vi "Main.vi"(11 "Module Admin":refnum<class "Delacor_lib_QMH_Module Admin.lvclass">) -> ()   [LabVIEW 2020, in "UI.lvlib"]
doc: "This template is based off of the Queued Message Handler design pattern and the Queued Message Handler project template that ships with LabVIEW.\n\nThe main difference is that the queue is private to this module and communication between modules is performed via Broadcast and Request events.\n\nRequest events are wrapped in public API methods and are handled in the Event Handling Loop (EHL) of this VI. Any module can register for Broadcast events sent by this module. The EHL generates messages based on user interface actions.\n\nThe Message Handling Loop (MHL) processes messages generated by the EHL, or by other messages. The messages are string values, so new messages can be added easily to the Message Cases case structure in the MHL. Each message cluster can also provide an optional value for Message Data, which is a variant that can be converted to whatever message-specific data is required.\n_____\nBased on Delacor QMH Project Template 5.0.0.82."
uses:
  UI.lvlib
  <vilib>/Delacor/Delacor QMH/Libraries/Module Admin_class/Delacor_lib_QMH_Module Admin.lvclass
  Module Data--cluster.ctl
  Stop Argument--cluster.ctl
  <vilib>/Delacor/Delacor QMH/Libraries/Message Queue_class/Delacor_lib_QMH_Message Queue.lvclass/Delacor_lib_QMH_Message Queue.ctl
  <vilib>/Delacor/Delacor QMH/Libraries/Module Admin_class/Delacor_lib_QMH_Module Admin.lvclass/Delacor_lib_QMH_Module Admin.ctl
  <vilib>/Delacor/Delacor QMH/Libraries/Message Queue_class/Delacor_lib_QMH_Enqueue Message (Single).vi
  <vilib>/Delacor/Delacor QMH/Libraries/Module Admin_class/Delacor_lib_QMH_Get External Launch.vi
  <vilib>/Utility/error.llb/Error Cluster From Error Code.vi
  <vilib>/ErrorRing/Error Ring.xnode
  <vilib>/Delacor/Delacor QMH/Libraries/Message Queue_class/Delacor_lib_QMH_Message Queue.lvclass
  Acquisiton Oscar Template/Acquisiton Oscar Template.lvlib
  Config/Config.lvlib
  Logging/Logging.lvlib
panel:
  in  "Config":bool
  in  "Stop Acq":bool
  in  "Start Acq":bool
  out "error out":errorcluster
  out "Status":string
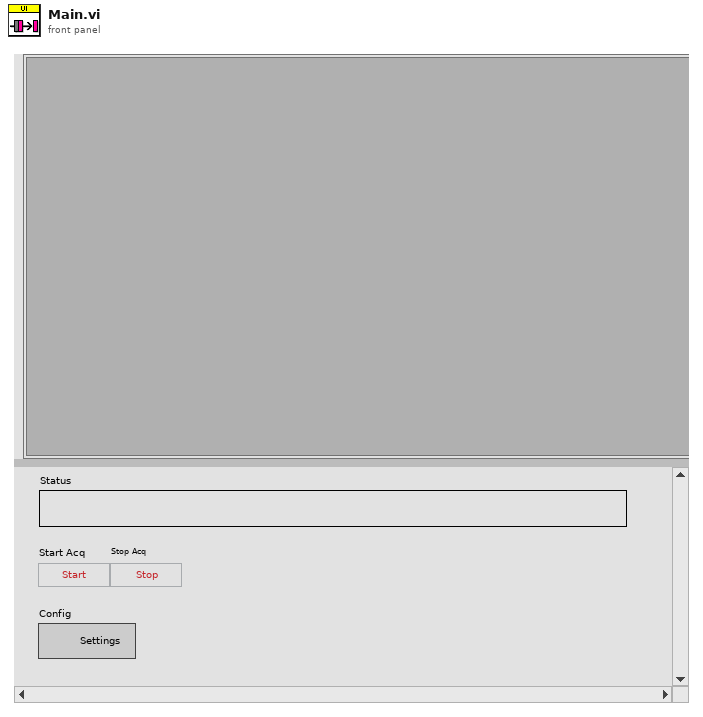
[diagram p1: front panel]
types:
  T1 = typedef "UI.lvlib/Request Events--cluster.ctl" = cluster{"Stop Module":refnum<user-event>, "Show Panel":refnum<user-event>, "Hide Panel":refnum<user-event>, "Get Module Execution Status":refnum<user-event>, "Show Diagram":refnum<user-event>}
  T2 = typedef "Acquisiton Oscar Template.lvlib/Broadcast Events--cluster.ctl" = cluster{"Module Did Init":refnum<user-event>, "Status Updated":refnum<user-event>, "Error Reported":refnum<user-event>, "Module Did Stop":refnum<user-event>, "Update Module Execution Status":refnum<user-event>}
  T3 = typedef "Config.lvlib/Broadcast Events--cluster.ctl" = cluster{"Module Did Init":refnum<user-event>, "Status Updated":refnum<user-event>, "Error Reported":refnum<user-event>, "Module Did Stop":refnum<user-event>, "Update Module Execution Status":refnum<user-event>}
  T4 = typedef "Logging.lvlib/Broadcast Events--cluster.ctl" = cluster{"Module Did Init":refnum<user-event>, "Status Updated":refnum<user-event>, "Error Reported":refnum<user-event>, "Module Did Stop":refnum<user-event>, "Update Module Execution Status":refnum<user-event>}
  T5 = typedef "UI.lvlib/Module Data--cluster.ctl" = cluster{"Status":string}
  T6 = enum32{"invalid lock state", "Not Locked", "Locked (No Password)", "Password-protected"}
  T7 = typedef "UI.lvlib/Stop Argument--cluster.ctl" = cluster{"Origin":string, "Exit via Stop Module Req?":bool, "Wait for Module to stop?":bool}
  T8 = enum32{"Invalid", "Standard", "Closed", "Hidden", "Minimized", "Maximized"}
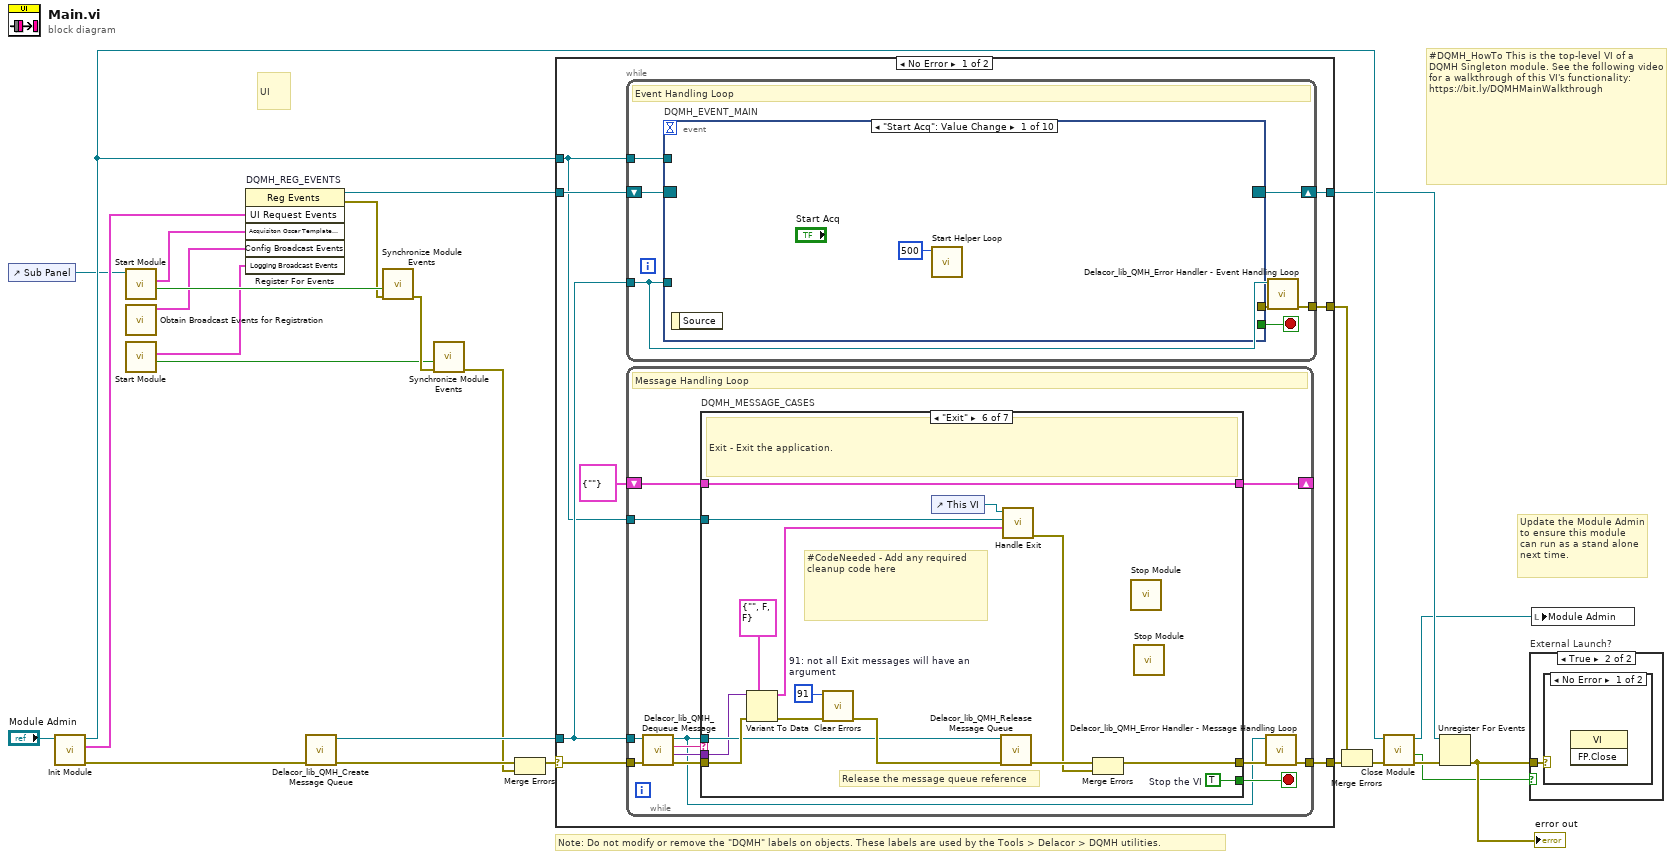
[diagram p0: block diagram]
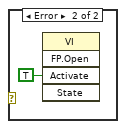
[diagram p3: hidden frame]
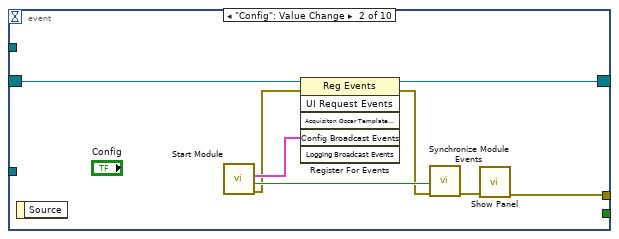
[diagram p4: hidden frame]
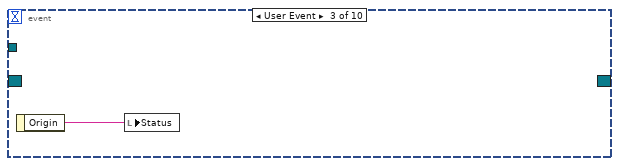
[diagram p5: hidden frame]
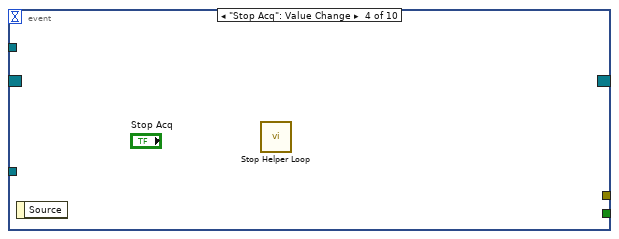
[diagram p6: hidden frame]
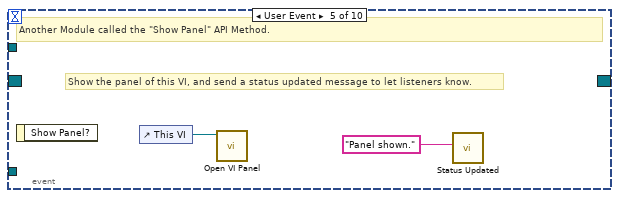
[diagram p7: hidden frame]
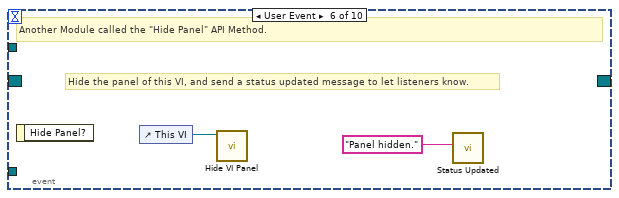
[diagram p8: hidden frame]
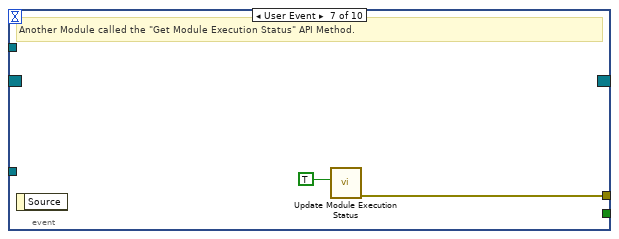
[diagram p9: hidden frame]
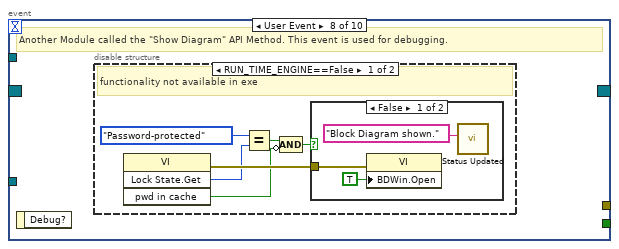
[diagram p10: hidden frame]
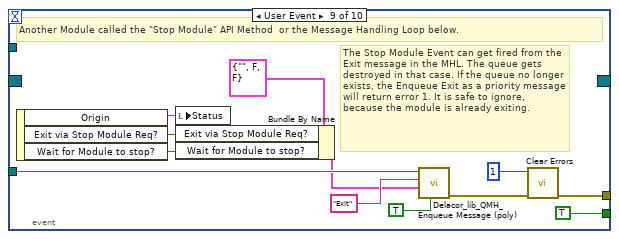
[diagram p13: hidden frame]
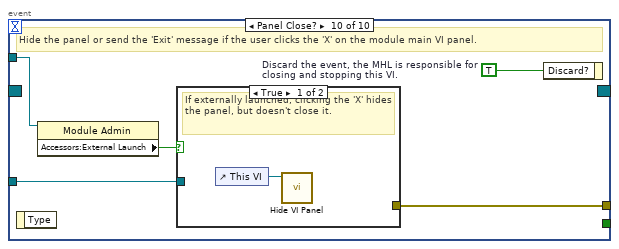
[diagram p14: hidden frame]
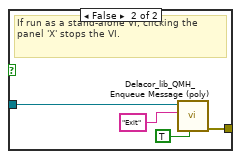
[diagram p15: hidden frame]
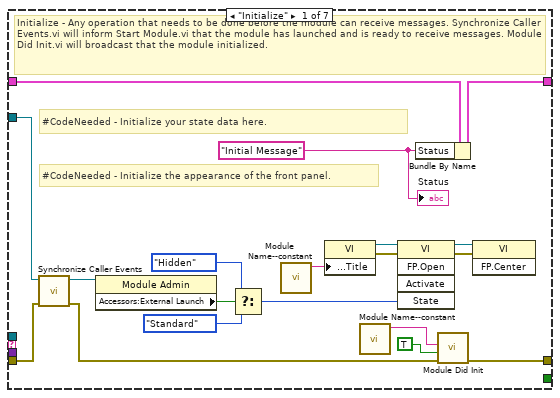
[diagram p16: hidden frame]
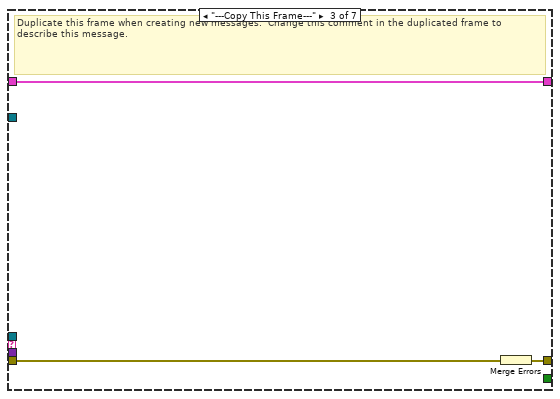
[diagram p18: hidden frame]
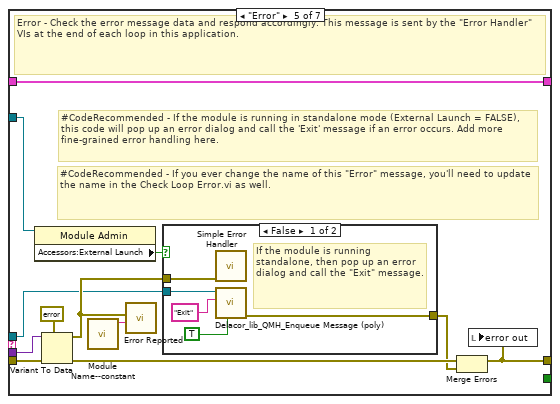
[diagram p20: hidden frame]
diagram:
  # "UI"
  # "#DQMH_HowTo This is the top-level VI of a DQMH Singleton module. See the following video for a walkthrough of this VI's functionality: https://bit.ly/DQMHMainWalkthrough"
  # "Note: Do not modify or remove the \"DQMH\" labels on objects. These labels are used by the Tools > Delacor > DQMH utilities."
  # "Update the Module Admin to ensure this module can run as a stand alone next time."
  n1 = control-ref of="Sub Panel"() -> (w6:refnum<vi>)
  n2 = call "Init Module.vi"("Singleton Module Admin in"="Module Admin") -> ("error out"=w24:errorcluster, "UI Request Events"=w14:T1, "Singleton Module Admin out"=w17:refnum<class "Delacor_lib_QMH_Module Admin.lvclass">)  [unwired: 8 in]
  n3 = call "Start Module.vi"("Sub Panel"=w6) -> ("Wait for Event Sync?"=w8:bool, "Acquisiton Oscar Template Broadcast Events"=w9:T2)  [unwired: 7 in, 2 out]
  n4 = call "Obtain Broadcast Events for Registration.vi"() -> ("Config Broadcast Events"=w5:T3)  [unwired: 9 in, 2 out]
  n5 = call "Start Module.vi"() -> ("Wait for Event Sync?"=w1:bool, "Logging Broadcast Events"=w2:T4)  [unwired: 8 in, 2 out]
  n6 = register-events "DQMH_REG_EVENTS"(w14, w9, w5, w2) -> (reference out=w15:refnum<event-registration>, error out=w7:errorcluster)  [unwired: 2 in]
  n7 = call <vilib>:"Delacor_lib_QMH_Create Message Queue.vi"("error in (no error)"=w24) -> ("error out"=w19:errorcluster, "Message Queue"=w13:refnum<class "Delacor_lib_QMH_Message Queue.lvclass">)  [unwired: 9 in]
  n8 = call "Synchronize Module Events.vi"("error in (no error)"=w7, "Wait for Event Sync?"=w8) -> ("error out"=w4:errorcluster)  [unwired: 9 in]
  n9 = call "Synchronize Module Events.vi"("error in (no error)"=w4, "Wait for Event Sync?"=w1) -> ("error out"=w3:errorcluster)  [unwired: 9 in]
  n10 = Merge Errors(w19, w3) -> (w18:errorcluster)
  n11 = case shown="No Error" w18 {
    selector: w18 -> [w31 w174]
    tunnel: [w33 w173] -> w25
    tunnel: [w30 w179] -> w16
    tunnel: w15 -> [w28 w179]
    tunnel: w13 -> [w27 w172]
    tunnel: [w32 _] -> w22
    tunnel: w17 -> [w26 w175]
    frame No Error {
      n12 = while {
        tunnel: w27 -> [w34]
        shift-right: [w37] -> w30
        shift-left: w28 -> [w38]
        tunnel: [w39] -> w32
        tunnel: w26 -> [w35]
        stop <- w36 stop-if-true
        # "Event Handling Loop"
        n13 = event "DQMH_EVENT_MAIN" shown="[0] \"Start Acq\": Value Change" {
          selector: w38 -> [_ w49 _ _ _ _ _ _ _ _]
          dyn-events: [_ w44 _ _ _ _ _ _ _ _] -> w37
          timeout: _ -> [_ _ _ _ _ _ _ _ _ _]
          tunnel: [_ _ _ _ _ _ _ _ TRUE ("Discard?") _] -> w36
          tunnel: w34 -> [_ _ _ _ _ _ _ _ w73 w80]
          tunnel: [_ w42 _ _ _ _ w56 _ w76 w82] -> w40
          tunnel: w35 -> [_ _ _ _ _ _ _ _ _ w79]
          event "Start Acq": Value Change {
            n14 = event-data() -> ()  [unwired: 1 in, 1 out]
            n15 = call "Start Helper Loop.vi"("Delay Timeout"=500) -> ()  [unwired: 10 in, 1 out]
          }
          event "Config": Value Change {
            n16 = event-data() -> ()  [unwired: 1 in, 1 out]
            n17 = call "Start Module.vi"() -> ("error out"=w46:errorcluster, "Wait for Event Sync?"=w47:bool, "Config Broadcast Events"=w48:T3)  [unwired: 8 in, 1 out]
            n18 = register-events(reference=w49, error in=w46, w48) -> (reference out=w44:refnum<event-registration>, error out=w45:errorcluster)  [unwired: 3 in]
            n19 = call "Synchronize Module Events.vi"("error in (no error)"=w45, "Wait for Event Sync?"=w47) -> ("error out"=w43:errorcluster)  [unwired: 9 in]
            n20 = call "Show Panel.vi"("error in (no error)"=w43) -> ("error out"=w42:errorcluster)  [unwired: 10 in]
          }
          event User Event {
            n21 = event-data() -> ("Origin"=w50:string)  [unwired: 1 in]
            n22 = local write "Status"(w50) -> ()
          }
          event "Stop Acq": Value Change {
            n23 = event-data() -> ()  [unwired: 1 in, 1 out]
            n24 = call "Stop Helper Loop.vi"() -> ()  [unwired: 11 in, 1 out]
          }
          event User Event {
            # "Show the panel of this VI, and send a status updated message to let listeners know."
            # "Another Module called the \"Show Panel\" API Method."
            n25 = event-data() -> ()  [unwired: 1 in, 1 out]
            n26 = control-ref of="This VI"() -> (w52:refnum<vi>)
            n27 = call "Open VI Panel.vi"("VI"=w52) -> ()  [unwired: 10 in, 1 out]
            n28 = call "Status Updated.vi"("Status"="Panel shown." ("format string")) -> ()  [unwired: 10 in, 1 out]
          }
          event User Event {
            # "Hide the panel of this VI, and send a status updated message to let listeners know."
            # "Another Module called the \"Hide Panel\" API Method."
            n29 = event-data() -> ()  [unwired: 1 in, 1 out]
            n30 = control-ref of="This VI"() -> (w54:refnum<vi>)
            n31 = call "Hide VI Panel.vi"("VI"=w54) -> ()  [unwired: 10 in, 1 out]
            n32 = call "Status Updated.vi"("Status"="Panel hidden." ("format string")) -> ()  [unwired: 10 in, 1 out]
          }
          event User Event {
            # "Another Module called the \"Get Module Execution Status\" API Method."
            n33 = event-data() -> ()  [unwired: 1 in, 1 out]
            n34 = call "Update Module Execution Status.vi"("Running?"=TRUE) -> ("error out"=w56:errorcluster)  [unwired: 10 in]
          }
          event User Event {
            # "Another Module called the \"Show Diagram\" API Method. This event is used for debugging."
            n35 = event-data() -> ()  [unwired: 1 in, 1 out]
            n36 = disable-structure shown="RUN_TIME_ENGINE==False" {
              frame condition #0 (active) {
                # "functionality not available in exe"
                n37 = invoke class="VI" method="Lock State.Get"() -> (error out=w62:errorcluster, "Get Lock State"=w61:T6, "pwd in cache"=w58:bool)  [unwired: 4 in, 1 out]
                n38 = Equal?(x=T6."Password-protected", y=w61) -> (x = y?=w59:bool)
                n39 = Compound Arithmetic op=AND(w59, invert w58) -> (w57:bool)
                n40 = case shown="False" w57 {
                  tunnel: w62 -> [w65 _]
                  frame False {
                    n41 = property class="VI"(error in=w65, "BDWin.Open"=TRUE ("Block Diagram Window:Open")) -> ()  [unwired: 1 in, 2 out]
                    n42 = call "Status Updated.vi"("Status"="Block Diagram shown." ("format string")) -> ()  [unwired: 10 in, 1 out]
                  }
                  frame True {
                    # "Password-protected VI, and the password is not in the cache. Do not show the diagram."
                  }
                }
              }
              frame condition #1 {
              }
            }
          }
          event User Event {
            # "The Stop Module Event can get fired from the Exit message in the MHL. The queue gets destroyed in that case. If the queue no longer exists, the Enqueue Exit as a priority message will return error 1. It is safe to ignore, because the module is already exiting."
            # "Another Module called the \"Stop Module\" API Method  or the Message Handling Loop below."
            n43 = event-data() -> ("Origin"=w72:string, "Exit via Stop Module Req?"=w68:bool, "Wait for Module to stop?"=w67:bool)  [unwired: 1 in]
            n44 = local write "Status"(w72) -> ()
            n45 = Bundle By Name(cluster=T7 {"Origin"="", "Exit via Stop Module Req?"=FALSE, "Wait for Module to stop?"=FALSE} ("Stop Argument"), "Exit via Stop Module Req?"=w68, "Wait for Module to stop?"=w67) -> (w66:T7)
            n46 = call-poly <vilib>:"Delacor_lib_QMH_Enqueue Message (poly).vi"("Priority Message? (F)"=TRUE, "Message Data"=w66, "Message"="Exit", "Message Queue in"=w73) -> ("error out"=w77:errorcluster)  [unwired: 6 in, 1 out]
            n47 = call <vilib>:"Clear Errors.vi"("error in (no error)"=w77, "specific error code to clear (0: all)"=1) -> ("error out"=w76:errorcluster)  [unwired: 4 in, 1 out]
          }
          event Panel Close? {
            w81 = TRUE  # Discard the event, the MHL is responsible for closing and stopping this VI.
            # "Hide the panel or send the 'Exit' message if the user clicks the 'X' on the module main VI panel."
            n48 = event-data() -> ()  [unwired: 1 in, 1 out]
            n49 = property class="Module Admin"(reference=w79) -> ("Accessors:External Launch"=w78:bool)  [unwired: 1 in, 2 out]
            n50 = case shown="True" w78 {
              tunnel: w80 -> [_ w86]
              tunnel: [_ w87] -> w82
              frame True {
                # "If externally launched, clicking the 'X' hides the panel, but doesn't close it."
                n51 = control-ref of="This VI"() -> (w83:refnum<vi>)
                n52 = call "Hide VI Panel.vi"("VI"=w83) -> ()  [unwired: 10 in, 1 out]
              }
              frame False {
                # "If run as a stand-alone VI, clicking the panel 'X' stops the VI."
                n53 = call-poly <vilib>:"Delacor_lib_QMH_Enqueue Message (poly).vi"("Priority Message? (F)"=TRUE, "Message"="Exit", "Message Queue in"=w86) -> ("error out"=w87:errorcluster)  [unwired: 7 in, 1 out]
              }
            }
            n54 = event-data("Discard?"=w81) -> ()  [unwired: 1 in, 1 out]
          }
        }
        n55 = call-dynamic "Delacor_lib_QMH_Error Handler - Event Handling Loop.vi"("error in (no error)"=w40, "Message Queue in"=w34) -> ("dup error in"=w39:errorcluster)  [unwired: 8 in, 1 out]
      }
      n56 = while {
        tunnel: w27 -> [w90]
        shift-right: [w94] -> _
        shift-left: T5 {"Status"=""} ("Data Cluster") -> [w95]
        tunnel: w31 -> [w98]
        tunnel: [w96] -> w33
        tunnel: w26 -> [w88]
        stop <- w93 stop-if-true
        # "Message Handling Loop"
        n57 = call-dynamic "Delacor_lib_QMH_Dequeue Message.vi"("error in (no error)"=w98, "Message Queue in"=w90) -> ("error out"=w97:errorcluster, "Message Data"=w91:variant, "Message"=w92:string, "Message Queue out"=w89:refnum<class "Delacor_lib_QMH_Message Queue.lvclass">)  [unwired: 6 in]
        n58 = case "DQMH_MESSAGE_CASES" shown="\"Exit\"" w92 {
          selector: w92 -> [_ _ _ _ _ _ w159]
          tunnel: w89 -> [_ _ _ _ w129 w151 _]
          tunnel: w97 -> [w116 w120 w123 w125 w136 w157 w161]
          tunnel: [w114 w120 w122 w125 w132 w154 w162] -> w99
          tunnel: w95 -> [w105 w119 w121 w124 w131 w150 w160]
          tunnel: [w104 w119 w121 w124 w131 w150 w160] -> w94
          tunnel: [_ _ _ _ _ w149 _] -> w93
          tunnel: w91 -> [_ _ _ _ w130 w148 _]
          tunnel: w88 -> [w106 _ _ _ w128 w143 _]
          frame "Initialize" {
            w100 = "Initial Message" ("Initial Message")
            # "#CodeNeeded - Initialize the appearance of the front panel."
            # "#CodeNeeded - Initialize your state data here."
            # "Initialize - Any operation that needs to be done before the module can receive messages. Synchronize Caller Events.vi will inform Start Module.vi that the module has launched and is ready to receive messages. Module Did Init.vi will broadcast that the module initialized."
            n59 = call "Synchronize Caller Events.vi"("error in (no error)"=w116, "Singleton Module Admin in"=w106) -> ("error out"=w115:errorcluster, "Singleton Module Admin out"=w101:refnum<class "Delacor_lib_QMH_Module Admin.lvclass">)  [unwired: 8 in]
            n60 = property class="Module Admin"(reference=w101) -> ("Accessors:External Launch"=w110:bool)  [unwired: 1 in, 2 out]
            n61 = Select(t=T8."Hidden" ("State"), s=w110, f=T8."Standard" ("State")) -> (s? t:f=w107:T8)
            n62 = call "Module Name--constant.vi"() -> ("Module Name"=w113:string)  [unwired: 11 in]
            n63 = property class="VI"("Front Panel.Title"=w113) -> (reference out=w112:refnum<vi>, error out=w118:errorcluster)  [unwired: 2 in]
            n64 = call "Module Name--constant.vi"() -> ("Module Name"=w102:string)  [unwired: 11 in]
            n65 = invoke class="VI" method="FP.Open"(reference=w112, error in=w118, "State"=w107) -> (reference out=w111:refnum<vi>, error out=w117:errorcluster)  [unwired: 2 in, 3 out]
            n66 = Bundle By Name(cluster=w105, "Status"=w100) -> (w104:T5)
            n67 = call "Module Did Init.vi"("error in (no error)"=w115, "Initialized?"=TRUE, "Origin"=w102) -> ("error out"=w114:errorcluster)  [unwired: 8 in]
            n68 = invoke class="VI" method="FP.Center"(reference=w111, error in=w117) -> ()  [unwired: 1 in, 3 out]
            "Status" <- w100
          }
          frame "--- Module Specific ---" {
            # "Separator -- The following cases handle messages specific to this Module."
          }
          frame "---Copy This Frame---" {
            # "Duplicate this frame when creating new messages.  Change this comment in the duplicated frame to describe this message."
            n69 = Merge Errors(w123) -> (w122:errorcluster)
          }
          frame "--- Exit and Error Handling---" {
            # "Separator - The following cases handle errors and exit messages."
          }
          frame "Error" {
            # "#CodeRecommended - If you ever change the name of this \"Error\" message, you'll need to update the name in the Check Loop Error.vi as well."
            # "#CodeRecommended - If the module is running in standalone mode (External Launch = FALSE), this code will pop up an error dialog and call the 'Exit' message if an error occurs. Add more fine-grained error handling here."
            # "Error - Check the error message data and respond accordingly. This message is sent by the \"Error Handler\" VIs at the end of each loop in this application."
            n70 = property class="Module Admin"(reference=w128) -> ("Accessors:External Launch"=w127:bool)  [unwired: 1 in, 2 out]
            n71 = Variant To Data(error in=w136, type=errorcluster {"status"=FALSE, "code"=0, "source"=""} ("error constant"), Variant=w130) -> (data=w137:errorcluster, error out=w134:errorcluster)
            n72 = call "Module Name--constant.vi"() -> ("Module Name"=w126:string)  [unwired: 11 in]
            n73 = call "Error Reported.vi"("Additional Information"=w126, "Error"=w137) -> ()  [unwired: 9 in, 1 out]
            n74 = case shown="False" w127 {
              tunnel: [w142 _] -> w133
              tunnel: w129 -> [w140 _]
              tunnel: w137 -> [w141 _]
              frame False {
                # "If the module is running standalone, then pop up an error dialog and call the \"Exit\" message."
                n75 = call <vilib>:"Simple Error Handler.vi"("error in (no error)"=w141) -> ()  [unwired: 4 in, 5 out]
                n76 = call-poly <vilib>:"Delacor_lib_QMH_Enqueue Message (poly).vi"("Priority Message? (F)"=TRUE, "Message"="Exit", "Message Queue in"=w140) -> ("error out"=w142:errorcluster)  [unwired: 7 in, 1 out]
              }
              frame True {
                # "If the module was launched externally, calling the Error Reported broadcast VI is the only action performed by the \"Error\" message. The module's caller can then process the error appropriately."
              }
            }
            n77 = Merge Errors(w134, w133) -> (w132:errorcluster)
            n78 = local write "error out"(w132) -> ()
          }
          frame "Exit" {
            w147 = 91  # 91: not all Exit messages will have an argument
            w149 = TRUE  # Stop the VI
            # "Release the message queue reference"
            # "#CodeNeeded - Add any required cleanup code here"
            # "Exit - Exit the application."
            n79 = Variant To Data(error in=w157, type=T7 {"Origin"="", "Exit via Stop Module Req?"=FALSE, "Wait for Module to stop?"=FALSE} ("Stop Argument"), Variant=w148) -> (data=w145:T7, error out=w153:errorcluster)
            n80 = call <vilib>:"Clear Errors.vi"("error in (no error)"=w153, "specific error code to clear (0: all)"=w147) -> ("error out"=w156:errorcluster)  [unwired: 4 in, 1 out]
            n81 = control-ref of="This VI"() -> (w144:refnum<vi>)
            n82 = call-dynamic "Delacor_lib_QMH_Release Message Queue.vi"("error in (no error)"=w156, "Message Queue"=w151) -> ("error out"=w155:errorcluster)  [unwired: 9 in]
            n83 = call "Handle Exit.vi"("Stop Argument"=w145, "Admin in"=w143, "VI reference"=w144) -> ("error out"=w152:errorcluster)  [unwired: 7 in, 1 out]
            n84 = Merge Errors(w155, w152) -> (w154:errorcluster)
            n85 = call "Stop Module.vi"() -> ()  [unwired: 11 in, 1 out]
            n86 = call "Stop Module.vi"() -> ()  [unwired: 11 in, 1 out]
          }
          frame Default {
            # "'Default' case only runs if there is a message that isn't defined in any of the other cases.  Output a programming error."
            n87 = call "Module Name--constant.vi"() -> ("Module Name"=w158:string)  [unwired: 11 in]
            n88 = xnode "Error Ring"("parameter 0"=w159, "parameter 1"=w158) -> ("error out"=w163:errorcluster)
            n89 = Merge Errors(w161, w163) -> (w162:errorcluster)
          }
        }
        n90 = call-dynamic "Delacor_lib_QMH_Error Handler - Message Handling Loop.vi"("error in (no error)"=w99, "Message Queue in"=w89) -> ("dup error in"=w96:errorcluster)  [unwired: 8 in, 1 out]
      }
    }
    frame Error {
      # "Synchronize Caller Events.vi will inform Start Module.vi that the module has launched and will let the code calling Start Module.vi register for broadcasts and would permit the caller receive the broadcast that an error occurred at launch time."
      n91 = call-dynamic "Delacor_lib_QMH_Release Message Queue.vi"("error in (no error)"=w174, "Message Queue"=w172) -> ("error out"=w173:errorcluster)  [unwired: 9 in]
      n92 = call "Synchronize Caller Events.vi"("Singleton Module Admin in"=w175) -> ("error out"=w180:errorcluster)  [unwired: 9 in, 1 out]
      n93 = call "Module Name--constant.vi"() -> ("Module Name"=w178:string)  [unwired: 11 in]
      n94 = Format Into String(format string="An error occurred during initialization. %s is no longer running.", w178) -> (resulting string=w176:string)  [unwired: 2 in, 1 out]
      n95 = Merge Errors(w173, w180) -> (w181:errorcluster)
      n96 = call "Error Reported.vi"("Additional Information"=w176, "Error"=w181) -> ()  [unwired: 9 in, 1 out]
    }
  }
  n97 = Merge Errors(w22, w25) -> (w21:errorcluster)
  n98 = call "Close Module.vi"("error in (no error)"=w21, "Module Admin in"=w17) -> ("error out"=w23:errorcluster, "External Launch"=w10:bool, "Module Admin out"=w11:refnum<class "Delacor_lib_QMH_Module Admin.lvclass">)  [unwired: 7 in]
  n99 = Unregister For Events(event registration refnum=w16, error in=w23) -> (error out=w20:errorcluster)
  "error out" <- w20
  n100 = case "External Launch?" shown="True" w10 {
    tunnel: w20 -> [_ w182]
    frame False {
    }
    frame True {
      n101 = case shown="No Error" w182 {
        frame No Error {
          n102 = invoke class="VI" method="FP.Close"() -> ()  [unwired: 3 in, 3 out]
        }
        frame Error {
          n103 = invoke class="VI" method="FP.Open"("Activate"=TRUE ("Activate?")) -> ()  [unwired: 4 in, 5 out]
        }
      }
    }
  }
  n104 = local write "Module Admin"(w11) -> ()
